vi "UI (Experienced).vi"() -> ()   [LabVIEW 2017, in "UI.lvlib"]
doc: "The Queued Message Handler of a Worker."
uses:
  UI.lvlib
  _support/Analysis Window Type.ctl
  _support/UI State.ctl
  1af51285-6659-428e-9c15-de70f1a207c9.vi
  1756710f-d813-4077-a3f9-6f06171a4225.vi
  b1498353-a107-4479-98d0-7e76c0451ff6.vi
  242d01f8-d211-4c25-bb6c-8191a2acbe42.vi
  da0d510b-1f54-4e49-9d1f-893e7e8abfcf.vi
  e403ca69-710b-4b23-8527-f02bfa86df9b.vi
  <userlib>/_NEVSTOP/Communicable State Machine(CSM)/AdvanceAPI/CSM - Revert Arguments-Safe String.vi
  <userlib>/_NEVSTOP/Communicable State Machine(CSM)/_Shared/Trim Single-line Text.vi
  <userlib>/_NEVSTOP/Communicable State Machine(CSM)/AdvanceAPI/CSM - Make String Arguments Safe.vi
  <userlib>/_NEVSTOP/Communicable State Machine(CSM)/AdvanceAPI/CSM - Break Down Multiple States String.vi
  <userlib>/_NEVSTOP/Communicable State Machine(CSM)/AdvanceAPI/CSM - Keywords.vi
  <userlib>/_NEVSTOP/Communicable State Machine(CSM)/addons/INI-Static-Variable-Support/_Support/instances/_CSM - Read File Logger Configuration - v1.0.vi
  <userlib>/_NEVSTOP/Communicable State Machine(CSM)/addons/API-String-Arugments-Support/_Support/Convert API String Arguments to Data(variant).vi
  <userlib>/_NEVSTOP/Communicable State Machine(CSM)/addons/API-String-Arugments-Support/_Support/Query Data as API String Arguments(variant).vi
  <userlib>/_NEVSTOP/Communicable State Machine(CSM)/addons/MassData-Parameter/_support/FGV-MassData(lvlibp).vi
  <userlib>/_NEVSTOP/Communicable State Machine(CSM)/_Polymophic/Add State(s) to Queue By BOOL(Element).vi
  <userlib>/_NEVSTOP/Communicable State Machine(CSM)/_Polymophic/CSM - Replace Marks in Messages.vi
  Acquisition/Acquisition.lvlib
  Logging/Logging.lvlib
  <userlib>/_NEVSTOP/Communicable State Machine(CSM)/Communicable State Machine.lvlib
  <userlib>/_NEVSTOP/Communicable State Machine(CSM)/addons/MassData-Parameter/CSM MassData Parameter Support.lvlib
  <userlib>/_NEVSTOP/Communicable State Machine(CSM)/addons/INI-Static-Variable-Support/INI-Static-Variable-Support.lvlib
  Algorithm/Algorithm.lvlib
  <userlib>/_NEVSTOP/Communicable State Machine(CSM)/addons/Logger/CSM File Logger.lvlib
  <userlib>/_NEVSTOP/Communicable State Machine(CSM)/addons/Watchdog/CSM Watchdog.lvlib
  <userlib>/_NEVSTOP/Communicable State Machine(CSM)/_Polymophic/Build Synchronous Message with Arguments.vi
panel:
  out "WaveformGraph":waveform(dbl)[](graph)
  in  "Analysis Window 1":T1
  out "AnalysisWnd 1":cluster{"f0":dbl, "df":dbl, "magnitude":dbl[]}[](graph)
  in  "Analysis Window 2":T1
  out "AnalysisWnd 2":cluster{"f0":dbl, "df":dbl, "magnitude":dbl[]}[](graph)
  in  "Settings":bool
  in  "Start":bool
  in  "Stop":bool
  out "Status":string
  in  "Exit":bool
  # "Continuous Measurement and Data Logger - CSM Version"
  # "Experienced Example"
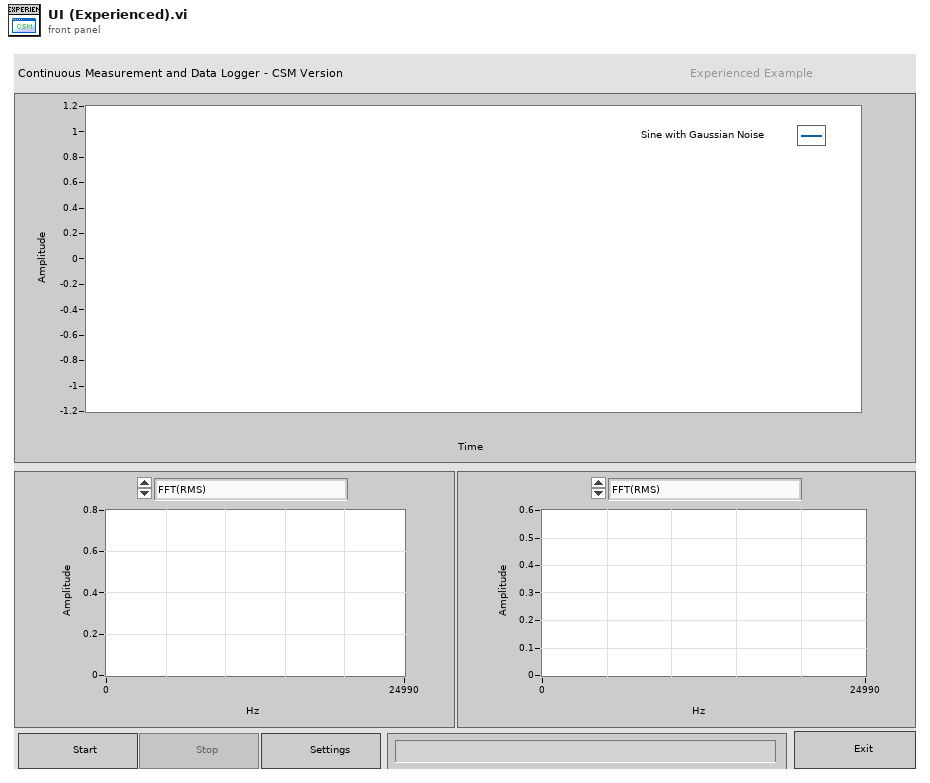
[diagram p1: front panel]
types:
  T1 = typedef "UI.lvlib/Analysis Window Type.ctl" = enum16{"FFT(RMS)", "FFT(Peak)", "Power Spectrum"}
  T2 = cluster{"Enable":bool, "Limit":cluster{"FileSize":i64, "FileNum":i32}, "Timestamp.Format":string, "AutoExit":bool}
  T3 = enum32{"Invalid", "Standard", "Closed", "Hidden", "Minimized", "Maximized"}
  T4 = enum32{"invalid app kind", "Development System", "Run Time System", "Student Edition", "Embedded LabVIEW", "Evaluation", "Custom"}
  T5 = typedef "UI.lvlib/UI State.ctl" = enum16{"Idle", "Acquiring and Logging", "Waiting for Exit", "Waiting for Exit (Acq Stopped)", "Waiting for Exit (Log Stopped)", "Waiting for Stop", "Waiting for Stop (Acq Stopped)", "Waiting for Stop (Log Stopped)"}
  T6 = enum32{"Invalid", "Default", "Floating", "Floating/Auto-Hide", "Modal"}
  T7 = typedef "Communicable State Machine.lvlib/_CSM_Response Source Message.ctl" = cluster{"‘State":string, "’Arguments":string, "’Error":errorcluster}
  T8 = cluster{"Current VI Reference":refnum<vi>, "Close Panel on Exit?":bool}
  T9 = cluster{"Core":cluster{"Current VI Reference":refnum<vi>, "Close Panel on Exit?":bool}, "UI Refs":cluster{"Start Ref":refnum<vi>, "Stop Ref":refnum<vi>, "Settings Ref":refnum<vi>, "Exit Ref":refnum<vi>, "Status Ref":refnum<vi>, "Data Ref":refnum<vi>, "Data Source Ref":refnum<vi>}, "State":T5, "Relationships":string}
  T10 = cluster{"Start Ref":refnum<vi>, "Stop Ref":refnum<vi>, "Settings Ref":refnum<vi>, "Exit Ref":refnum<vi>, "Status Ref":refnum<vi>, "Data Ref":refnum<vi>, "Data Source Ref":refnum<vi>}
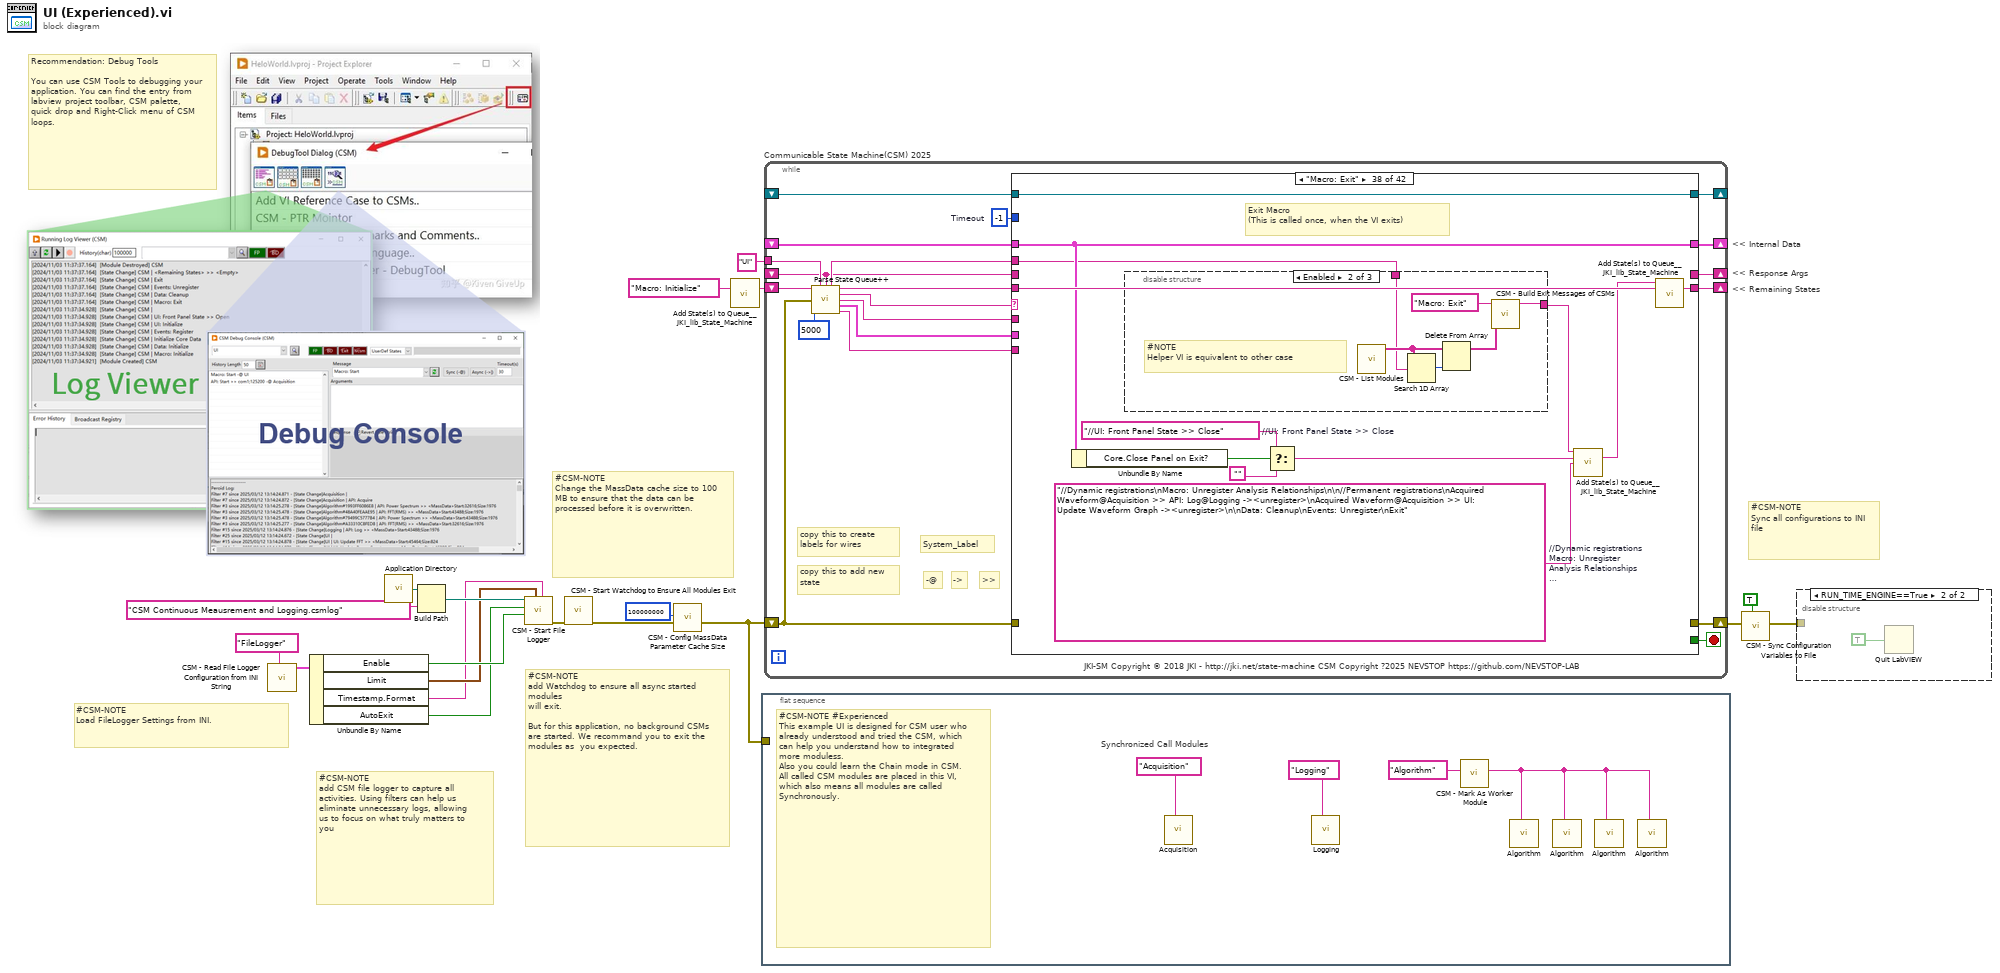
[diagram p0: block diagram]
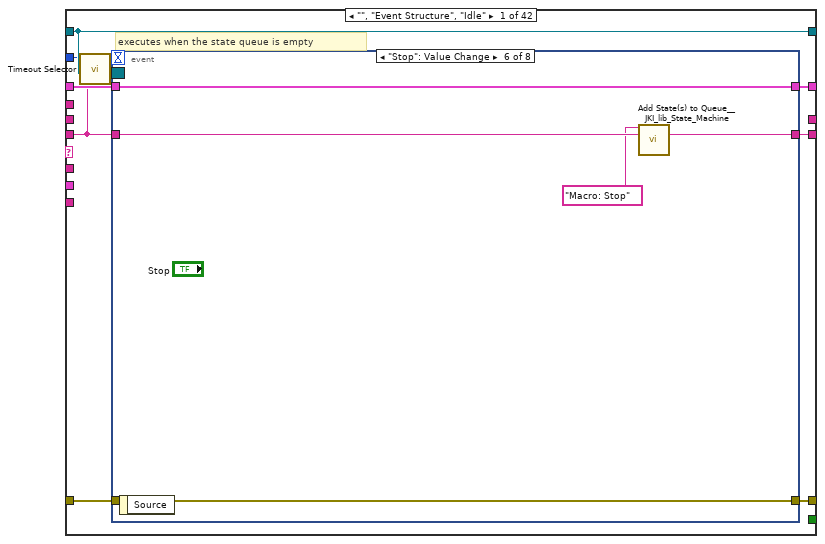
[diagram p3: hidden frame]
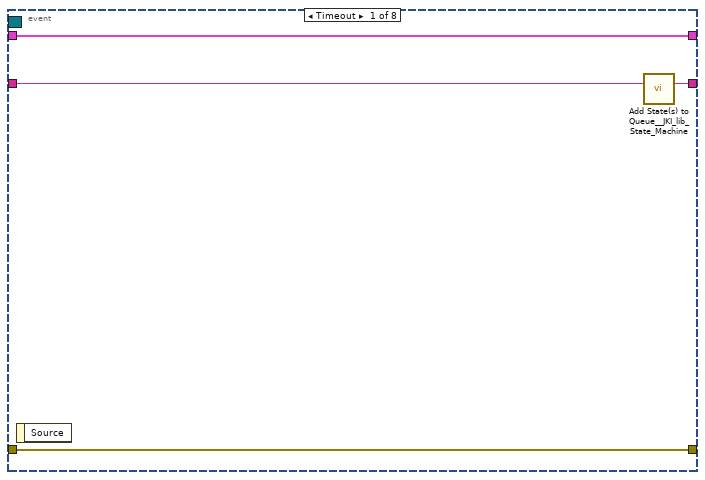
[diagram p4: hidden frame]
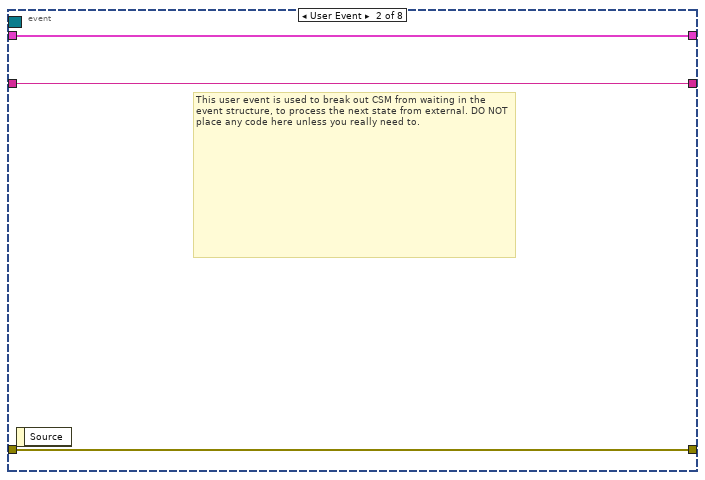
[diagram p5: hidden frame]
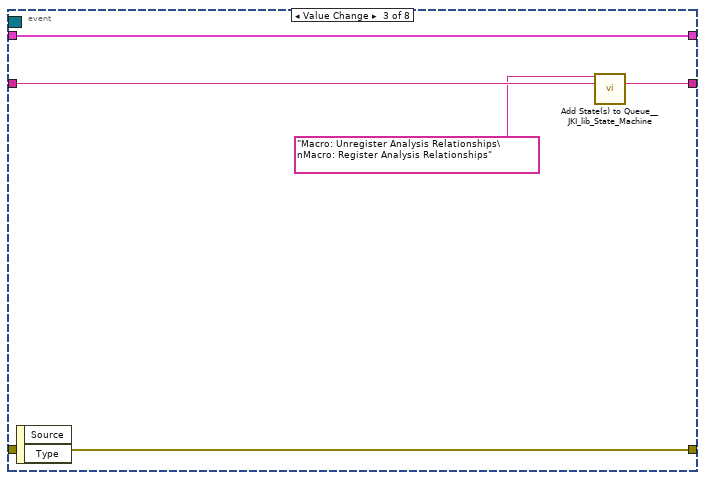
[diagram p6: hidden frame]
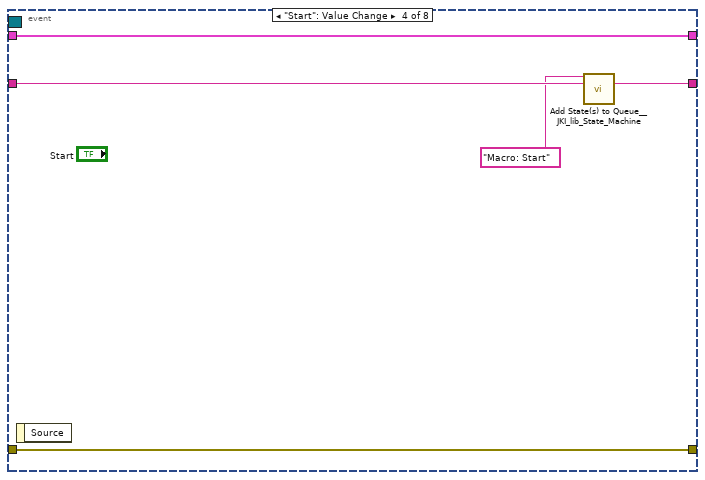
[diagram p7: hidden frame]
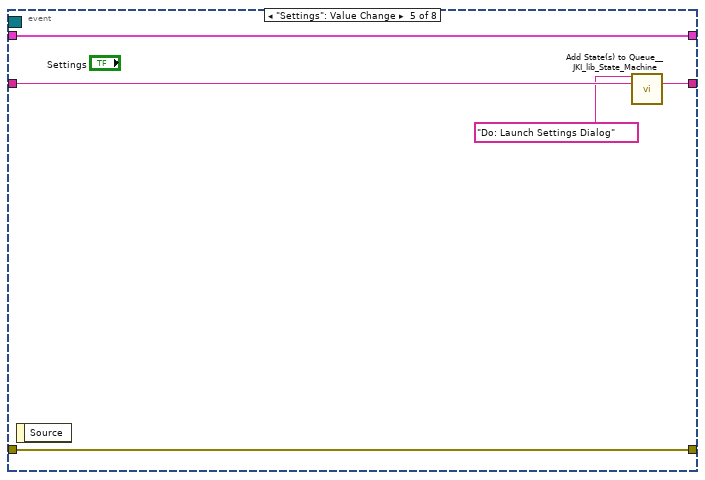
[diagram p8: hidden frame]
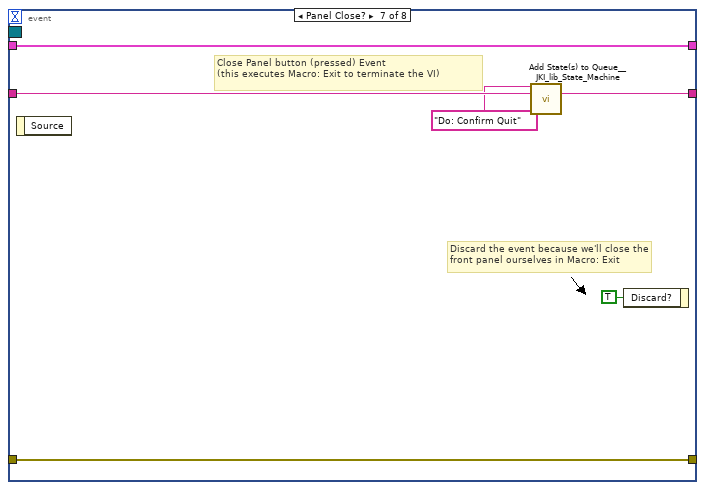
[diagram p9: hidden frame]
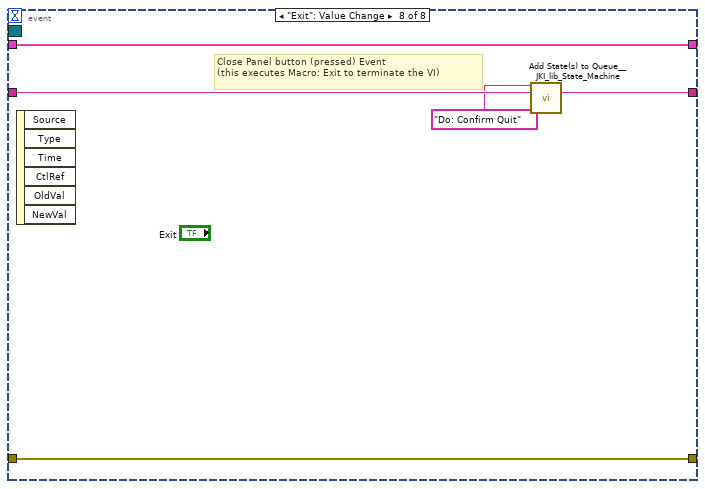
[diagram p10: hidden frame]
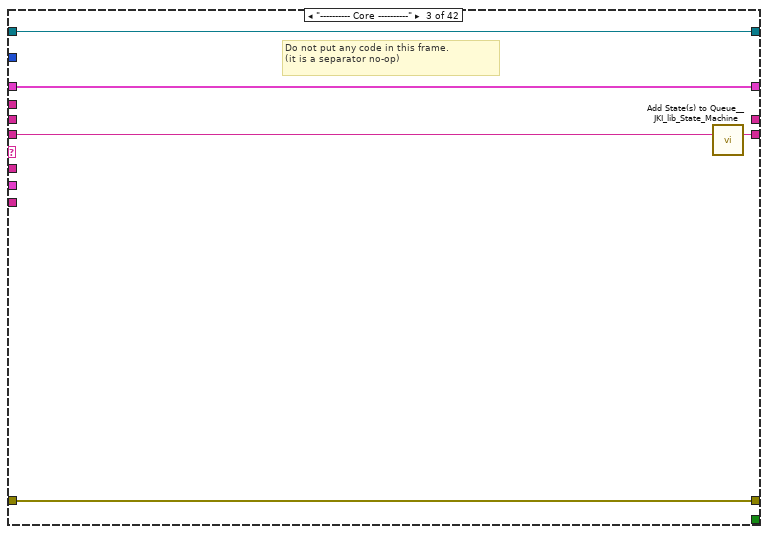
[diagram p12: hidden frame]
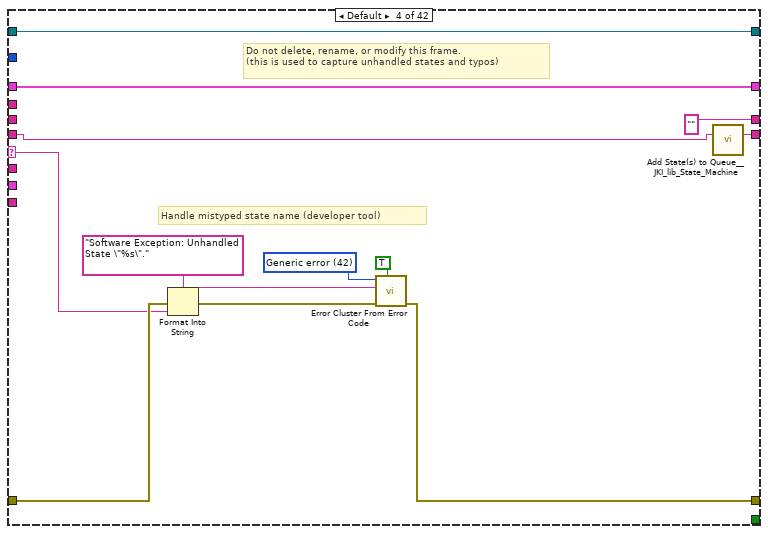
[diagram p13: hidden frame]
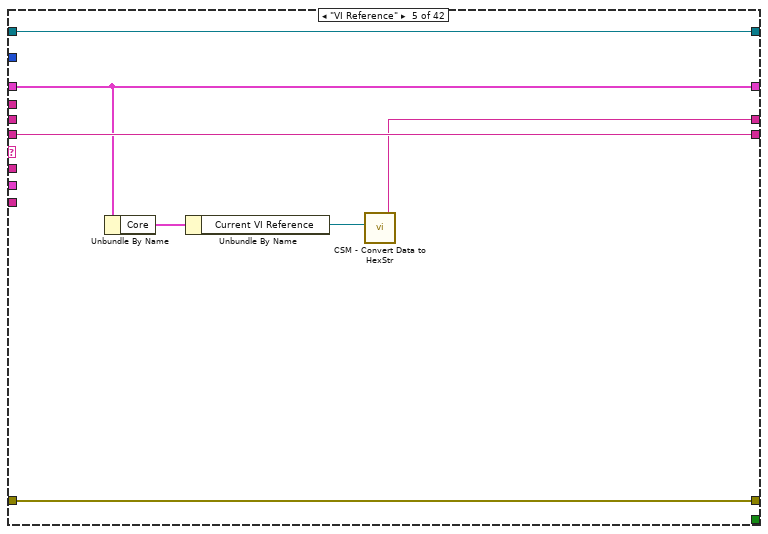
[diagram p14: hidden frame]
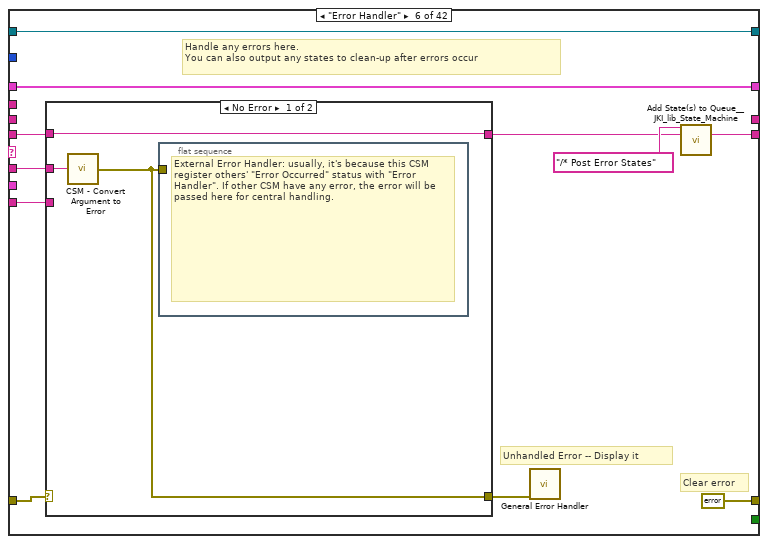
[diagram p15: hidden frame]
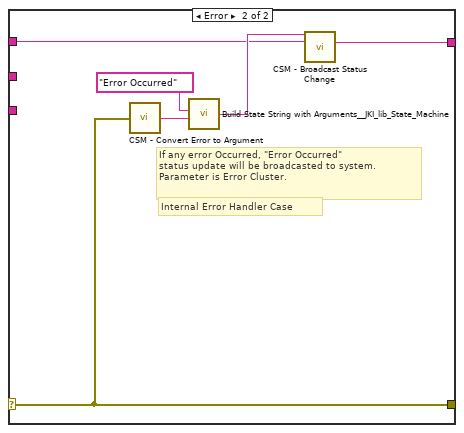
[diagram p16: hidden frame]
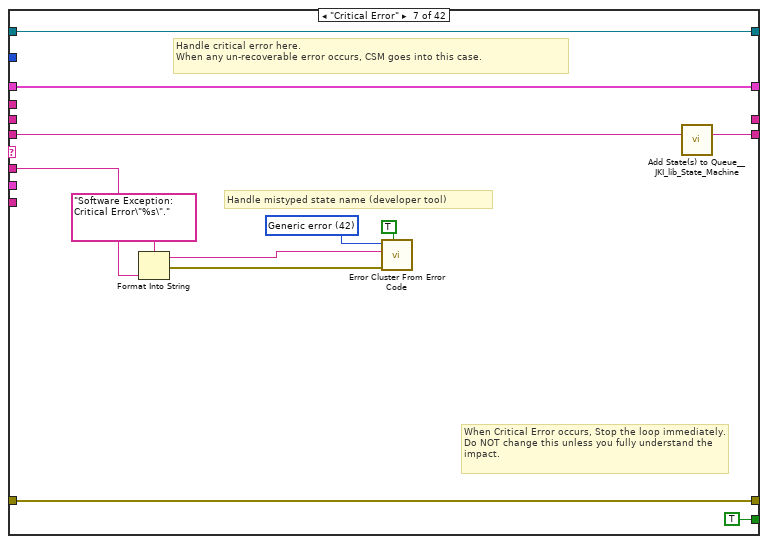
[diagram p17: hidden frame]
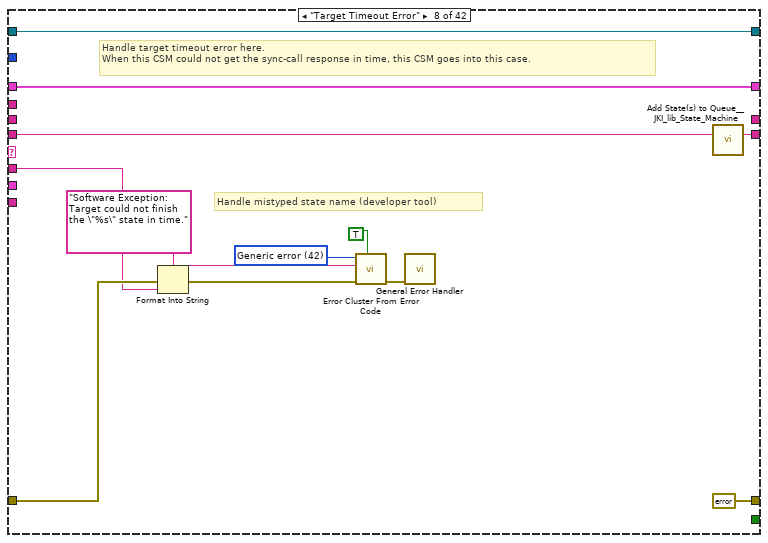
[diagram p18: hidden frame]
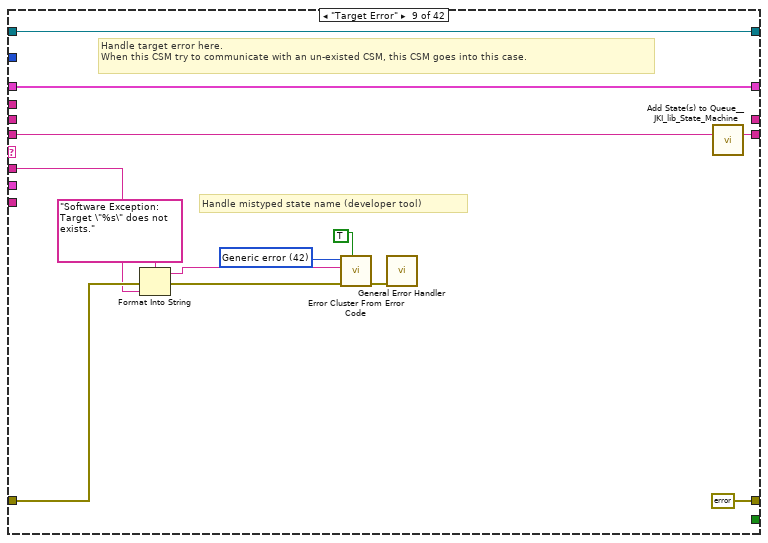
[diagram p19: hidden frame]
diagram:
  # "#CSM-NOTE\nSync all configurations to INI file"
  # "#CSM-NOTE\nChange the MassData cache size to 100 MB to ensure that the data can be processed before it is overwritten."
  # "Recommendation: Debug Tools\n\nYou can use CSM Tools to debugging your application. You can find the entry from labview project toolbar, CSM palette, quick drop and Right-Click menu of CSM loops."
  # "#CSM-NOTE\nLoad FileLogger Settings from INI."
  # "#CSM-NOTE\nadd CSM file logger to capture all activities. Using filters can help us eliminate unnecessary logs, allowing us to focus on what truly matters to you"
  # "#CSM-NOTE\nadd Watchdog to ensure all async started modules\nwill exit. \n\nBut for this application, no background CSMs are started. We recommand you to exit the modules as  you expected."
  # "<< Internal Data"
  # "<< Response Args"
  # "<< Remaining States"
  n1 = call-poly <userlib>:"CSM - Read File Logger Configuration from INI String.vi"("Section Name(\"FileLogger\")"="FileLogger" ("Section Name(\"\" as Default)")) -> ("FileLogger Configuration-v1"=w11:T2)  [unwired: 7 in, 1 out]
  n2 = Unbundle By Name(w11) -> ("Enable"=w10:bool, "Limit"=w9:cluster{"FileSize":i64, "FileNum":i32}, "Timestamp.Format"=w7:string, "AutoExit"=w8:bool)
  n3 = call <vilib>:"Application Directory.vi"() -> ("Application Directory"=w16:path)
  n4 = Build Path(base path=w16, name or relative path="CSM Continuous Meausrement and Logging.csmlog") -> (appended path=w14:path)
  n5 = call <userlib>:"CSM - Start File Logger.vi"("Timestamp Format"=w7, "Log Limit"=w9, "Watchdog? (T)"=w10, "Exit When All Module Exist? (F)"=w8, "Log File Path"=w14) -> ("error out"=w13:errorcluster)  [unwired: 4 in, 2 out]
  n6 = call <userlib>:"CSM - Start Watchdog to Ensure All Modules Exit.vi"("error in (no error)"=w13) -> ("error out"=w5:errorcluster)  [unwired: 10 in]
  n7 = call <userlib>:"CSM - Config MassData Parameter Cache Size.vi"("Error in"=w5, "Size (50M)"=100000000 ("size(1M)")) -> ("Error out"=w4:errorcluster)  [unwired: 9 in]
  n8 = call <vilib>:"Add State(s) to Queue__JKI_lib_State_Machine.vi"("State(s) in (\"\")"="Macro: Initialize") -> ("States Out"=w17:string)  [unwired: 14 in]
  n9 = flat-sequence {
    tunnel: w4 -> [_]
    frame #0 {
      # "#CSM-NOTE #Experienced\nThis example UI is designed for CSM user who already understood and tried the CSM, which can help you understand how to integrated more moduless.\nAlso you could learn the Chain mode in CSM.\nAll called CSM modules are placed in this VI, which also means all modules are called  Synchronously."
      # "Synchronized Call Modules"
      n10 = call "Acquisition.vi"("Name(\"\" to use uuid)"="Acquisition" ("Name(\"\" to use uuid)")) -> ()  [unwired: 11 in]
      n11 = call "Logging.vi"("Name(\"\" to use uuid)"="Logging" ("Name(\"\" to use uuid)")) -> ()  [unwired: 11 in]
      n12 = call <userlib>:"CSM - Mark As Worker Module.vi"("CSM Name"="Algorithm" ("Name(\"\" to use uuid)")) -> ("CSM Name (Marked As Worker)"=w21:string)  [unwired: 9 in]
      n13 = call "Algorithm.vi"("Name(\"\" to use uuid)"=w21) -> ()  [unwired: 11 in]
      n14 = call "Algorithm.vi"("Name(\"\" to use uuid)"=w21) -> ()  [unwired: 11 in]
      n15 = call "Algorithm.vi"("Name(\"\" to use uuid)"=w21) -> ()  [unwired: 11 in]
      n16 = call "Algorithm.vi"("Name(\"\" to use uuid)"=w21) -> ()  [unwired: 11 in]
    }
  }
  n17 = while "Communicable State Machine(CSM) 2025" {
    shift-right: [w39] -> _
    shift-left: _ -> [w38]
    shift-right: [w41] -> w2
    shift-left: w4 -> [w36]
    shift-right: [w40] -> _
    shift-left: w17 -> [w42]
    tunnel: "UI" ("Name(\"\" to use uuid)") -> [w31]
    shift-right: [w34] -> _
    shift-left: _ -> [w26]
    shift-right: [w33] -> _
    shift-left: _ -> [w32]
    stop <- w24 stop-if-true
    w37 = -1  # Timeout
    # "JKI-SM Copyright © 2018 JKI - http://jki.net/state-machine CSM Copyright ?2025 NEVSTOP https://github.com/NEVSTOP-LAB"
    # "copy this to add new state"
    # ">>"
    # "->"
    # "-@"
    # "copy this to create labels for wires"
    # "System_Label"
    n18 = call <userlib>:"Parse State Queue++.vi"("State Queue"=w42, "Name (\"\" to Use UUID)"=w31, "Response Arguments"=w26, "Previous Error"=w36, "Response Timeout (-2 Use Global Settings)"=5000 ("Response Timeout(1000ms)")) -> ("Name Used"=w27:string, "Remaining States"=w43:string, "Current State"=w30:string, "Arguments"=w25:string, "Additional Information"=w29:T7, "Source CSM"=w28:string)  [unwired: 5 in]
    n19 = case shown="\"Macro: Exit\"" w30 {
      selector: w30 -> [_ _ _ w102 _ _ _ _ _ _ _ _ _ _ _ _ _ _ _ _ _ _ _ _ _ _ _ _ _ _ _ _ _ _ _ _ _ _ _ _ _ _]
      tunnel: w43 -> [w44 w93 w99 w106 w118 w123 w149 w159 w172 w180 w184 w199 w206 w211 w220 w226 w233 w240 w245 w251 w255 w261 w281 w295 w308 w316 w332 w406 w415 w428 w435 w440 w447 w455 w463 w474 w485 w503 w528 w534 w542 w580]
      tunnel: w25 -> [_ _ _ _ _ w121 w142 w155 w168 _ _ _ _ _ _ w224 w230 _ _ _ _ _ _ _ _ w311 w326 w401 w419 w425 w432 _ _ _ _ _ _ _ _ w529 _ _]
      tunnel: w38 -> [w51 w92 w96 w104 w117 w129 w150 w157 w170 w179 w183 w192 w204 w208 _ w223 w231 w235 w242 w250 w254 w258 w267 w285 w298 w314 w328 w404 w421 w427 w434 w437 w444 w458 w470 w477 w481 w501 w525 w531 w535 w575]
      tunnel: [w50 w94 w97 w108 w119 errorcluster {"status"=FALSE, "code"=0, "source"=""} ("error out") w151 errorcluster {"status"=FALSE, "code"=0, "source"=""} ("error out") errorcluster {"status"=FALSE, "code"=0, "source"=""} ("error out") w181 w185 w196 w203 w209 w214 w222 w229 w236 w243 w246 w253 w259 w279 w296 w309 w312 w329 w398 w417 w424 w431 w438 w445 w459 w472 w480 w489 _ w526 w532 w536 _] -> w41
      tunnel: w36 -> [w49 w94 w97 w107 w119 w127 w151 w160 w173 w181 w185 w196 w203 w209 w214 _ _ w237 w243 _ w256 w259 w279 w296 w309 w313 w330 _ _ _ _ w438 w445 w459 w472 w480 w489 _ w526 w532 _ _]
      tunnel: [w52 w93 w98 w105 w118 w125 w148 w158 w171 w180 w184 w198 w205 w210 w219 w226 w233 w239 w244 w251 w255 w260 w280 w295 w308 w315 w331 w406 w416 w428 w435 w439 w446 w456 w464 w475 w486 w502 w527 w533 w542 w573] -> w40
      tunnel: [_ _ _ _ _ _ TRUE _ _ _ _ _ TRUE _ _ _ _ _ _ _ _ _ _ _ _ _ _ _ _ _ _ _ _ _ _ _ _ _ _ _ _ _] -> w24
      tunnel: [w48 w92 w96 w104 w117 w129 w150 w157 w170 w179 w183 w197 w204 w208 w213 w221 w227 w235 w242 w250 w254 w258 w266 w285 w298 w314 w328 w404 w421 w427 w434 w437 w444 w454 w461 w476 w487 w501 w525 w531 w535 w574] -> w39
      tunnel: w37 -> [w46 _ _ _ _ _ _ _ _ _ _ _ _ _ _ _ _ _ _ _ _ _ _ _ _ _ _ _ _ _ _ _ _ _ _ _ _ _ _ _ _ _]
      tunnel: w28 -> [_ _ _ _ _ w120 _ _ _ _ _ _ _ _ _ _ _ _ _ _ _ _ _ _ _ _ _ _ _ _ _ _ _ _ _ _ _ _ _ _ _ _]
      tunnel: w29 -> [_ _ _ _ _ _ _ _ _ _ _ _ _ _ _ _ _ _ _ _ _ _ _ _ _ _ _ _ _ _ _ _ _ _ _ _ _ _ _ _ _ _]
      tunnel: [_ _ _ "" w113 _ _ _ _ _ _ _ _ _ _ _ w228 _ _ _ _ _ _ _ _ _ _ _ _ _ _ _ _ _ _ _ _ _ _ _ _ _] -> w34
      tunnel: [w47 w91 w95 w100 w116 w128 w140 w154 w167 w178 w182 w186 w201 w207 w217 w225 w232 w234 w241 w249 w252 w257 w278 w294 w307 w310 w325 w405 w420 w426 w433 w436 w443 w457 w471 w479 w488 w494 w524 w530 w543 w579] -> w33
      tunnel: w32 -> [w47 w91 w95 w100 w116 w128 w140 w154 w167 w178 w182 w186 w201 w207 w217 w225 w232 w234 w241 _ w252 w257 w278 w294 w307 w310 w325 w405 w420 w426 w433 w436 w443 w457 w471 w479 w488 w494 w524 w530 w543 w579]
      tunnel: w27 -> [_ _ _ _ _ _ _ _ _ _ _ _ _ _ _ _ _ _ _ w248 _ _ _ _ _ _ _ _ _ _ _ _ _ _ _ _ _ w492 _ _ w538 _]
      tunnel: w26 -> [_ _ _ _ _ _ _ _ _ _ _ _ _ _ _ _ _ _ _ _ _ _ _ _ _ _ _ _ _ _ _ _ _ _ _ _ _ _ _ _ _ _]
      frame "", "Event Structure", "Idle" {
        # "executes when the state queue is empty"
        n20 = call <userlib>:"Timeout Selector.vi"("Remaining States"=w44, "Timeout Expected"=w46) -> ("Timeout"=w45:i32)  [unwired: 5 in]
        n21 = event shown="[5] \"Stop\": Value Change" {
          selector: w47 -> [_ _ _ _ _ _ _ _]
          dyn-events: _ -> [_ _ _ _ _ _ _ _]
          timeout: w45 -> [_ _ _ _ _ _ _ _]
          tunnel: w44 -> [w56 w58 w61 w66 w71 w76 w85 w90]
          tunnel: [w55 w58 w62 w67 w72 w77 w84 w89] -> w52
          tunnel: w51 -> [w53 w59 w63 w68 w73 w78 w82 w87]
          tunnel: [w54 w57 w64 w69 w74 w79 w83 w88] -> w50
          tunnel: w49 -> [w54 w57 w64 w69 w74 w79 w83 w88]
          tunnel: [w53 w59 w63 w68 w73 w78 w82 w87] -> w48
          event Timeout {
            n22 = event-data() -> ()  [unwired: 1 in, 1 out]
            n23 = call <vilib>:"Add State(s) to Queue__JKI_lib_State_Machine.vi"("State(s) in (\"\")"=w56) -> ("States Out"=w55:string)  [unwired: 14 in]
          }
          event User Event {
            # "This user event is used to break out CSM from waiting in the event structure, to process the next state from external. DO NOT place any code here unless you really need to."
            n24 = event-data() -> ()  [unwired: 1 in, 1 out]
          }
          event Value Change {
            n25 = event-data() -> ()  [unwired: 1 in, 2 out]
            n26 = call <vilib>:"Add State(s) to Queue__JKI_lib_State_Machine.vi"("State(s) in Front (\"\")"="Macro: Unregister Analysis Relationships\nMacro: Register Analysis Relationships" ("State(s) in Front (\"\")"), "State(s) in (\"\")"=w61) -> ("States Out"=w62:string)  [unwired: 13 in]
          }
          event "Start": Value Change {
            n27 = event-data() -> ()  [unwired: 1 in, 1 out]
            n28 = call <vilib>:"Add State(s) to Queue__JKI_lib_State_Machine.vi"("State(s) in Front (\"\")"="Macro: Start" ("State(s) in Front (\"\")"), "State(s) in (\"\")"=w66) -> ("States Out"=w67:string)  [unwired: 13 in]
          }
          event "Settings": Value Change {
            n29 = event-data() -> ()  [unwired: 1 in, 1 out]
            n30 = call <vilib>:"Add State(s) to Queue__JKI_lib_State_Machine.vi"("State(s) in Front (\"\")"="Do: Launch Settings Dialog" ("State(s) in Front (\"\")"), "State(s) in (\"\")"=w71) -> ("States Out"=w72:string)  [unwired: 13 in]
          }
          event "Stop": Value Change {
            n31 = event-data() -> ()  [unwired: 1 in, 1 out]
            n32 = call <vilib>:"Add State(s) to Queue__JKI_lib_State_Machine.vi"("State(s) in Front (\"\")"="Macro: Stop" ("State(s) in Front (\"\")"), "State(s) in (\"\")"=w76) -> ("States Out"=w77:string)  [unwired: 13 in]
          }
          event Panel Close? {
            # "Discard the event because we'll close the front panel ourselves in Macro: Exit"
            # "Close Panel button (pressed) Event\n(this executes Macro: Exit to terminate the VI)"
            n33 = event-data() -> ()  [unwired: 1 in, 1 out]
            n34 = call <vilib>:"Add State(s) to Queue__JKI_lib_State_Machine.vi"("State(s) in Front (\"\")"="Do: Confirm Quit", "State(s) in (\"\")"=w85) -> ("States Out"=w84:string)  [unwired: 13 in]
            n35 = event-data("Discard?"=TRUE) -> ()  [unwired: 1 in, 1 out]
          }
          event "Exit": Value Change {
            # "Close Panel button (pressed) Event\n(this executes Macro: Exit to terminate the VI)"
            n36 = event-data() -> ()  [unwired: 1 in, 6 out]
            n37 = call <vilib>:"Add State(s) to Queue__JKI_lib_State_Machine.vi"("State(s) in Front (\"\")"="Do: Confirm Quit", "State(s) in (\"\")"=w90) -> ("States Out"=w89:string)  [unwired: 13 in]
          }
        }
      }
      frame "CSM Documentation" {
        # "CSM Documentation"
        # "State Syntax:\nStateCategory: State >> Argument -@ CSMName\nStateCategory: State >> Argument -> CSMName\n\nLine Terminator: Line feed"
        # "Commenting:\nTo add a comment use \"//\" or \"#\" and all text to the right will be ignored\nCommenting Example:\nUI: Initialize // This initializes the UI\n// Another comment line"
        # "Example:\nUI: Help >> About -@Main\nUI: Help >> About ->Main\n\nWhere \"UI\" is the state category\nWhere \"Help\" is the state\nWhere \"About\" is the argument\nWhere \"Main\" is the Name of CSM,which actually run the \"UI: Help >> About\"\n\n    \"-@\" stands for sync state. Current CSM will wait until the state is finished. \n            - if \"Main\" named CSM does not exist, \"Target Error\" will occur.\n            - if \"Main\" named CSM is in another sync remote state, \"Target Busy Error\" will occur.\n            - if \"Main\" named CSM could not finish the state in time, \"Target Timeout Error\" will occur.\n            - if everything is right. \"Response\" will occur with Argument back from \"Main\" named CSM. \n\n    \"->\" stands for async state. Current CSM will post the state and continue to next state in next iteration.\n            - if \"Main\" named CSM does not exist, \"Target Error\" will occur.\n            - if everything is right. \"Async Message Posted\" will occur.\n            - After State is finished. Caller will receive a \"Async Response\" state from callee.\n\nWhen duplicated name is used for multiple CSM module or some framework problem happens, \"Critical Error\" will occur."
      }
      frame "---------- Core ----------" {
        # "Do not put any code in this frame.\n(it is a separator no-op)"
        n38 = call <vilib>:"Add State(s) to Queue__JKI_lib_State_Machine.vi"("State(s) in (\"\")"=w99) -> ("States Out"=w98:string)  [unwired: 14 in]
      }
      frame Default {
        w111 = 42 items=["No error", "Argument error", "Memory is full", "Out of zone", "End of file", "File already open", "Generic file I/O error", "File not found", "File permission error", "Disk is full", "Duplicate path", "Too many files open", "System feature not enabled", "Resource file not found", "Cannot add resource", "Resource not found", "Image not found", "Image memory error", "Pen does not exist", "Config type invalid", "Config token not found", "Config parse error", "Config memory error", "Bad external code format", "Bad external code offset", "External code not present", "Null window", "Destroy window error", "Null menu", "Print aborted", "Bad print record", "Print driver error", "Windows error during printing", "Memory error during printing", "Print dialog error", "Generic print error", "Invalid device refnum", "Device not found", "Device parameter error", "Device unit error", "Cannot open device", "Device call aborted", "Generic error", "Cancelled by user", "Object ID too low", "Object ID too high", "Object not in heap", "Unknown heap", "Unknown object (invalid DefProc)", "Unknown object (DefProc not in table)", "Message out of range", "Invalid (null) method", "Unknown message", "Manager call not supported", "Bad address", "Network operation in progress", "Network operation timed out", "Connection is busy", "Network attribute not supported", "Network error", "Address in use", "System out of memory", "Connection aborted", "Connection refused", "Not connected", "Already connected", "Connection closed", "Initialization error (interapplication manager)", "Bad occurrence", "Wait on unbound occurrence handler", "Occurrence queue overflow", "Datalog type conflict", "Unused", "Unrecognized type (interapplication manager)", "Memory corrupt", "Failed to make temporary DLL", "Old CIN version", "Drag socket not found", "Failed to load drop-object", "Failed to register OLE object", "Failed to release OLE object", "Format specifier type mismatch", "Unknown format specifier", "Too few format specifiers", "Too many format specifiers", "Scan failed", "Newer CIN version", "Error converting to variant", "Runtime menu error", "Password tampered", "Variant attribute not found", "Incompatible variant data type", "Event data is not available", "Event Store is not present", "Occurrence is not found", "Event Queue is not created", "Event info is not available", "Refnum passed is NULL", "Error retrieving Class GUID", "Error retrieving CoClass GUID", "Error retrieving TypeLib GUID.", "Bad built application magic bytes.", "Specific driver is different from the specific driver associated with the Logical Name.", "There is no session opened to the class driver.", "Max Error", "MAX - Error with config objects", "MAX - Error loading configuration", "MAX - Group not supported"]
        # "Do not delete, rename, or modify this frame.\n(this is used to capture unhandled states and typos)"
        # "Handle mistyped state name (developer tool)"
        n39 = Format Into String(format string="Software Exception: Unhandled State \"%s\"." ("message"), error in=w107, w102) -> (resulting string=w110:string, error out=w109:errorcluster)  [unwired: 1 in]
        n40 = call <vilib>:"Error Cluster From Error Code.vi"("show call chain? (False)"=TRUE, "error in (no error)"=w109, "error message (\"\")"=w110, "error code (0)"=w111) -> ("error out"=w108:errorcluster)  [unwired: 5 in]
        n41 = call <vilib>:"Add State(s) to Queue__JKI_lib_State_Machine.vi"("State(s) in (\"\")"=w106) -> ("States Out"=w105:string)  [unwired: 14 in]
      }
      frame "VI Reference" {
        n42 = Unbundle By Name(w117) -> ("Core"=w115:T8)
        n43 = Unbundle By Name(w115) -> ("Current VI Reference"=w114:refnum<vi>)
        n44 = call <userlib>:"CSM - Convert Data to HexStr.vi"("Variant"=w114) -> ("HEX String (0-9,A-F)"=w113:string)  [unwired: 8 in]
      }
      frame "Error Handler" {
        # "Unhandled Error -- Display it"
        # "Handle any errors here.\nYou can also output any states to clean-up after errors occur"
        # "Clear error"
        n45 = case shown="No Error" w127 {
          selector: w127 -> [_ w134]
          tunnel: [w132 w136] -> w124
          tunnel: w123 -> [w132 w135]
          tunnel: [w131 w134] -> w122
          tunnel: w121 -> [w133 _]
          tunnel: w120 -> [_ _]
          frame No Error {
            n46 = call <userlib>:"CSM - Convert Argument to Error.vi"("Argument"=w133) -> ("Error"=w131:errorcluster)  [unwired: 4 in]
            n47 = flat-sequence {
              tunnel: w131 -> [_]
              frame #0 {
                # "External Error Handler: usually, it's because this CSM register others' \"Error Occurred\" status with \"Error Handler\". If other CSM have any error, the error will be passed here for central handling."
              }
            }
          }
          frame Error {
            # "Internal Error Handler Case"
            # "If any error Occurred, \"Error Occurred\" \nstatus update will be broadcasted to system.\nParameter is Error Cluster."
            n48 = call <userlib>:"CSM - Convert Error to Argument.vi"("Error"=w134) -> ("Argument"=w138:string)  [unwired: 4 in]
            n49 = call <vilib>:"Build State String with Arguments__JKI_lib_State_Machine.vi"("Arguments (\"\")"=w138, "State"="Error Occurred" ("Status with Arguments")) -> ("State with Arguments"=w137:string)  [unwired: 4 in]
            n50 = call <userlib>:"CSM - Broadcast Status Change.vi"("Status With Arguments"=w137, "State Queue"=w135) -> ("Remaining States"=w136:string)  [unwired: 13 in]
          }
        }
        n51 = call <vilib>:"General Error Handler.vi"("error in (no error)"=w122) -> ()  [unwired: 10 in, 5 out]
        n52 = call <vilib>:"Add State(s) to Queue__JKI_lib_State_Machine.vi"("State(s) in Front (\"\")"="/* Post Error States", "State(s) in (\"\")"=w124) -> ("States Out"=w125:string)  [unwired: 13 in]
      }
      frame "Critical Error" {
        w146 = 42 items=["No error", "Argument error", "Memory is full", "Out of zone", "End of file", "File already open", "Generic file I/O error", "File not found", "File permission error", "Disk is full", "Duplicate path", "Too many files open", "System feature not enabled", "Resource file not found", "Cannot add resource", "Resource not found", "Image not found", "Image memory error", "Pen does not exist", "Config type invalid", "Config token not found", "Config parse error", "Config memory error", "Bad external code format", "Bad external code offset", "External code not present", "Null window", "Destroy window error", "Null menu", "Print aborted", "Bad print record", "Print driver error", "Windows error during printing", "Memory error during printing", "Print dialog error", "Generic print error", "Invalid device refnum", "Device not found", "Device parameter error", "Device unit error", "Cannot open device", "Device call aborted", "Generic error", "Cancelled by user", "Object ID too low", "Object ID too high", "Object not in heap", "Unknown heap", "Unknown object (invalid DefProc)", "Unknown object (DefProc not in table)", "Message out of range", "Invalid (null) method", "Unknown message", "Manager call not supported", "Bad address", "Network operation in progress", "Network operation timed out", "Connection is busy", "Network attribute not supported", "Network error", "Address in use", "System out of memory", "Connection aborted", "Connection refused", "Not connected", "Already connected", "Connection closed", "Initialization error (interapplication manager)", "Bad occurrence", "Wait on unbound occurrence handler", "Occurrence queue overflow", "Datalog type conflict", "Unused", "Unrecognized type (interapplication manager)", "Memory corrupt", "Failed to make temporary DLL", "Old CIN version", "Drag socket not found", "Failed to load drop-object", "Failed to register OLE object", "Failed to release OLE object", "Format specifier type mismatch", "Unknown format specifier", "Too few format specifiers", "Too many format specifiers", "Scan failed", "Newer CIN version", "Error converting to variant", "Runtime menu error", "Password tampered", "Variant attribute not found", "Incompatible variant data type", "Event data is not available", "Event Store is not present", "Occurrence is not found", "Event Queue is not created", "Event info is not available", "Refnum passed is NULL", "Error retrieving Class GUID", "Error retrieving CoClass GUID", "Error retrieving TypeLib GUID.", "Bad built application magic bytes.", "Specific driver is different from the specific driver associated with the Logical Name.", "There is no session opened to the class driver.", "Max Error", "MAX - Error with config objects", "MAX - Error loading configuration", "MAX - Group not supported"]
        # "Handle critical error here.\nWhen any un-recoverable error occurs, CSM goes into this case."
        # "When Critical Error occurs, Stop the loop immediately. Do NOT change this unless you fully understand the impact."
        # "Handle mistyped state name (developer tool)"
        n53 = Format Into String(format string="Software Exception: Critical Error\"%s\"." ("message"), w142) -> (resulting string=w145:string, error out=w144:errorcluster)  [unwired: 2 in]
        n54 = call <vilib>:"Error Cluster From Error Code.vi"("show call chain? (False)"=TRUE, "error in (no error)"=w144, "error message (\"\")"=w145, "error code (0)"=w146) -> ()  [unwired: 5 in, 1 out]
        n55 = call <vilib>:"Add State(s) to Queue__JKI_lib_State_Machine.vi"("State(s) in (\"\")"=w149) -> ("States Out"=w148:string)  [unwired: 14 in]
      }
      frame "Target Timeout Error" {
        w163 = 42 items=["No error", "Argument error", "Memory is full", "Out of zone", "End of file", "File already open", "Generic file I/O error", "File not found", "File permission error", "Disk is full", "Duplicate path", "Too many files open", "System feature not enabled", "Resource file not found", "Cannot add resource", "Resource not found", "Image not found", "Image memory error", "Pen does not exist", "Config type invalid", "Config token not found", "Config parse error", "Config memory error", "Bad external code format", "Bad external code offset", "External code not present", "Null window", "Destroy window error", "Null menu", "Print aborted", "Bad print record", "Print driver error", "Windows error during printing", "Memory error during printing", "Print dialog error", "Generic print error", "Invalid device refnum", "Device not found", "Device parameter error", "Device unit error", "Cannot open device", "Device call aborted", "Generic error", "Cancelled by user", "Object ID too low", "Object ID too high", "Object not in heap", "Unknown heap", "Unknown object (invalid DefProc)", "Unknown object (DefProc not in table)", "Message out of range", "Invalid (null) method", "Unknown message", "Manager call not supported", "Bad address", "Network operation in progress", "Network operation timed out", "Connection is busy", "Network attribute not supported", "Network error", "Address in use", "System out of memory", "Connection aborted", "Connection refused", "Not connected", "Already connected", "Connection closed", "Initialization error (interapplication manager)", "Bad occurrence", "Wait on unbound occurrence handler", "Occurrence queue overflow", "Datalog type conflict", "Unused", "Unrecognized type (interapplication manager)", "Memory corrupt", "Failed to make temporary DLL", "Old CIN version", "Drag socket not found", "Failed to load drop-object", "Failed to register OLE object", "Failed to release OLE object", "Format specifier type mismatch", "Unknown format specifier", "Too few format specifiers", "Too many format specifiers", "Scan failed", "Newer CIN version", "Error converting to variant", "Runtime menu error", "Password tampered", "Variant attribute not found", "Incompatible variant data type", "Event data is not available", "Event Store is not present", "Occurrence is not found", "Event Queue is not created", "Event info is not available", "Refnum passed is NULL", "Error retrieving Class GUID", "Error retrieving CoClass GUID", "Error retrieving TypeLib GUID.", "Bad built application magic bytes.", "Specific driver is different from the specific driver associated with the Logical Name.", "There is no session opened to the class driver.", "Max Error", "MAX - Error with config objects", "MAX - Error loading configuration", "MAX - Group not supported"]
        # "Handle target timeout error here.\nWhen this CSM could not get the sync-call response in time, this CSM goes into this case."
        # "Handle mistyped state name (developer tool)"
        n56 = Format Into String(format string="Software Exception: Target could not finish the \"%s\" state in time." ("message"), error in=w160, w155) -> (resulting string=w162:string, error out=w161:errorcluster)  [unwired: 1 in]
        n57 = call <vilib>:"Error Cluster From Error Code.vi"("show call chain? (False)"=TRUE, "error in (no error)"=w161, "error message (\"\")"=w162, "error code (0)"=w163) -> ("error out"=w152:errorcluster)  [unwired: 5 in]
        n58 = call <vilib>:"General Error Handler.vi"("error in (no error)"=w152) -> ()  [unwired: 10 in, 5 out]
        n59 = call <vilib>:"Add State(s) to Queue__JKI_lib_State_Machine.vi"("State(s) in (\"\")"=w159) -> ("States Out"=w158:string)  [unwired: 14 in]
      }
      frame "Target Error" {
        w176 = 42 items=["No error", "Argument error", "Memory is full", "Out of zone", "End of file", "File already open", "Generic file I/O error", "File not found", "File permission error", "Disk is full", "Duplicate path", "Too many files open", "System feature not enabled", "Resource file not found", "Cannot add resource", "Resource not found", "Image not found", "Image memory error", "Pen does not exist", "Config type invalid", "Config token not found", "Config parse error", "Config memory error", "Bad external code format", "Bad external code offset", "External code not present", "Null window", "Destroy window error", "Null menu", "Print aborted", "Bad print record", "Print driver error", "Windows error during printing", "Memory error during printing", "Print dialog error", "Generic print error", "Invalid device refnum", "Device not found", "Device parameter error", "Device unit error", "Cannot open device", "Device call aborted", "Generic error", "Cancelled by user", "Object ID too low", "Object ID too high", "Object not in heap", "Unknown heap", "Unknown object (invalid DefProc)", "Unknown object (DefProc not in table)", "Message out of range", "Invalid (null) method", "Unknown message", "Manager call not supported", "Bad address", "Network operation in progress", "Network operation timed out", "Connection is busy", "Network attribute not supported", "Network error", "Address in use", "System out of memory", "Connection aborted", "Connection refused", "Not connected", "Already connected", "Connection closed", "Initialization error (interapplication manager)", "Bad occurrence", "Wait on unbound occurrence handler", "Occurrence queue overflow", "Datalog type conflict", "Unused", "Unrecognized type (interapplication manager)", "Memory corrupt", "Failed to make temporary DLL", "Old CIN version", "Drag socket not found", "Failed to load drop-object", "Failed to register OLE object", "Failed to release OLE object", "Format specifier type mismatch", "Unknown format specifier", "Too few format specifiers", "Too many format specifiers", "Scan failed", "Newer CIN version", "Error converting to variant", "Runtime menu error", "Password tampered", "Variant attribute not found", "Incompatible variant data type", "Event data is not available", "Event Store is not present", "Occurrence is not found", "Event Queue is not created", "Event info is not available", "Refnum passed is NULL", "Error retrieving Class GUID", "Error retrieving CoClass GUID", "Error retrieving TypeLib GUID.", "Bad built application magic bytes.", "Specific driver is different from the specific driver associated with the Logical Name.", "There is no session opened to the class driver.", "Max Error", "MAX - Error with config objects", "MAX - Error loading configuration", "MAX - Group not supported"]
        # "Handle target error here.\nWhen this CSM try to communicate with an un-existed CSM, this CSM goes into this case."
        # "Handle mistyped state name (developer tool)"
        n60 = Format Into String(format string="Software Exception: Target \"%s\" does not exists." ("message"), error in=w173, w168) -> (resulting string=w175:string, error out=w174:errorcluster)  [unwired: 1 in]
        n61 = call <vilib>:"Error Cluster From Error Code.vi"("show call chain? (False)"=TRUE, "error in (no error)"=w174, "error message (\"\")"=w175, "error code (0)"=w176) -> ("error out"=w166:errorcluster)  [unwired: 5 in]
        n62 = call <vilib>:"General Error Handler.vi"("error in (no error)"=w166) -> ()  [unwired: 10 in, 5 out]
        n63 = call <vilib>:"Add State(s) to Queue__JKI_lib_State_Machine.vi"("State(s) in (\"\")"=w172) -> ("States Out"=w171:string)  [unwired: 14 in]
      }
      frame "Async Response", "Response" {
        # "Handle Async-call Response (\"Async Response\" for ->)"
        # "Handle Sync-call Response (\"Response\" for -@)"
        # "After Message is executed, CSM+ goes to this state for receive the response. \n    For Async Message(->), \"Async Response\" is used. This CSM will goes to \"Async Message Posted\" immediately and receive the \"Async Response\" after the callee finishes the message.\n    For Sync Message(@),  This CSM will wait until the message is done and immediately goes to \"Response\""
      }
      frame "Async Message Posted" {
        # "Handle post action for async message (->)."
        # "After Async Message is posted (->), CSM+ goes to this state for post-action. You can use Argument - State to tell which Async Message is called."
      }
      frame "Initialize Core Data" {
        # "Do not delete, rename, or modify this frame.\n(this is used to determine panel behavior on exit)"
        # "originally closed?"
        # "exe?"
        # "If panel starts closed or is an EXE, then close it when we exit"
        n64 = property class="VI"() -> ("FP.State"=w189:T3)  [unwired: 2 in, 2 out]
        n65 = property class="App"() -> ("App.Kind"=w195:T4)  [unwired: 2 in, 2 out]
        n66 = control-ref of="Current VI Reference"() -> (w190:refnum<vi>)
        n67 = Equal?(x=w189, y=T3."Closed" ("Front Panel Window:State")) -> (x = y?=w187:bool)
        n68 = Equal?(x=w195, y=T4."Run Time System" ("Application:Kind")) -> (x = y?=w193:bool)
        n69 = Or(x=w187, y=w193) -> (x .or. y?=w191:bool)
        n70 = Bundle By Name(cluster=w192, "Core.Current VI Reference"=w190, "Core.Close Panel on Exit?"=w191) -> (w197:T9)
        n71 = call <vilib>:"Add State(s) to Queue__JKI_lib_State_Machine.vi"("State(s) in (\"\")"=w199) -> ("States Out"=w198:string)  [unwired: 14 in]
      }
      frame "Exit" {
        # "Do not put any code in this frame.\n(No errors that occur here will be handled.)"
        n72 = local write "Status"("Exit" ("Exit String")) -> ()
        n73 = call <vilib>:"Add State(s) to Queue__JKI_lib_State_Machine.vi"("State(s) in (\"\")"=w206) -> ("States Out"=w205:string)  [unwired: 14 in]
      }
      frame "---------- Data ----------" {
        # "Do not put any code in this frame.\n(It is a separator no-op. You can make a copy of this frame to create a new Data frame)"
        n74 = call <vilib>:"Add State(s) to Queue__JKI_lib_State_Machine.vi"("State(s) in (\"\")"=w211) -> ("States Out"=w210:string)  [unwired: 14 in]
      }
      frame "Data: Initialize" {
        w212 = ""  # Relationships
        w215 = UI_State."Idle"  # State
        w216 = T10 {"Start Ref"=refnum, "Stop Ref"=refnum, "Settings Ref"=refnum, "Exit Ref"=refnum, "Status Ref"=refnum, "Data Ref"=refnum, "Data Source Ref"=refnum}  # UI Refs
        w218 = T8 {"Current VI Reference"=refnum, "Close Panel on Exit?"=FALSE}  # Core
        # "Initialize the shift-register data, here.\n(data names are defined by what you wire into the bundle function)"
        n75 = Bundle("Core"=w218, "UI Refs"=w216, "State"=w215, "Relationships"=w212) -> (w213:T9)  [unwired: 1 in]
        n76 = call <vilib>:"Add State(s) to Queue__JKI_lib_State_Machine.vi"("State(s) in (\"\")"=w220) -> ("States Out"=w219:string)  [unwired: 14 in]
      }
      frame "Data: Set Configuration" {
        n77 = call "Convert API String Arguments to Data.vim"("Reference Type"=w223, "API String"=w224) -> ("error out"=w222:errorcluster, "Data"=w221:T9)  [unwired: 6 in]
      }
      frame "Data: Get Configuration", "Data: Get Internal Data" {
        n78 = call "Query Data as API String Arguments.vim"("Name"=w230, "Cluster Data"=w231) -> ("error"=w229:errorcluster, "API String"=w228:string, "Cluster Data (dup)"=w227:T9)  [unwired: 7 in]
      }
      frame "Data: Cleanup" {
        # "Cleanup any data and references, here.\n(this is called automatically, by the Macro: Exit)"
        n79 = Unbundle By Name(w235) -> ("Core.Current VI Reference"=w238:refnum<vi>)
        n80 = Close Reference(reference=w238, error in (no error)=w237) -> (error out=w236:errorcluster)
        n81 = call <vilib>:"Add State(s) to Queue__JKI_lib_State_Machine.vi"("State(s) in (\"\")"=w240) -> ("States Out"=w239:string)  [unwired: 14 in]
      }
      frame "---------- Events ----------" {
        # "Do not put any code in this frame.\n(It is a separator no-op. You can make a copy of this frame to create a new UI frame)"
        n82 = call <vilib>:"Add State(s) to Queue__JKI_lib_State_Machine.vi"("State(s) in (\"\")"=w245) -> ("States Out"=w244:string)  [unwired: 14 in]
      }
      frame "Events: Register" {
        # "Register message event to break Waiting in Event structure."
        n83 = call <userlib>:"CSM - Get New State Notifier Event.vi"("Name (\"\" to Use UUID)"=w248) -> ("error out"=w246:errorcluster, "New State Notifier Event"=w247:refnum<user-event>)  [unwired: 9 in]
        n84 = register-events(w247) -> (reference out=w249:refnum<event-registration>)  [unwired: 2 in, 1 out]
      }
      frame "Events: Unregister" {
        n85 = Unregister For Events(event registration refnum=w252, error in=w256) -> (error out=w253:errorcluster)
      }
      frame "---------- UI ----------" {
        # "Do not put any code in this frame.\n(It is a separator no-op. You can make a copy of this frame to create a new UI frame)"
        n86 = call <vilib>:"Add State(s) to Queue__JKI_lib_State_Machine.vi"("State(s) in (\"\")"=w261) -> ("States Out"=w260:string)  [unwired: 14 in]
      }
      frame "UI: Initialize" {
        w262 = cluster{"f0":dbl, "df":dbl, "magnitude":dbl[]}[] [] ("FFT")
        # "Initialize the User Interface, here.\n(this is called automatically, by the Macro: Init)"
        n87 = control-ref of="WaveformGraph"() -> (w270:refnum<vi>)
        n88 = property on="AnalysisWnd 1" class="WFGraph (strict)"("Value"=w262) -> ()  [unwired: 2 in, 2 out]
        n89 = property on="AnalysisWnd 2" class="WFGraph (strict)"("Value"=w262) -> ()  [unwired: 2 in, 2 out]
        n90 = property on="WaveformGraph" class="WFChart (strict)"("History Data"=waveform(dbl)[][] []) -> ()  [unwired: 2 in, 2 out]
        n91 = control-ref of="Start"() -> (w275:refnum<vi>)
        n92 = control-ref of="Stop"() -> (w274:refnum<vi>)
        n93 = control-ref of="Settings"() -> (w276:refnum<vi>)
        n94 = control-ref of="Exit"() -> (w277:refnum<vi>)
        n95 = control-ref of="Status"() -> (w271:refnum<vi>)
        n96 = Bundle By Name(cluster=w267, "UI Refs.Start Ref"=w275, "UI Refs.Stop Ref"=w274, "UI Refs.Settings Ref"=w276, "UI Refs.Exit Ref"=w277, "UI Refs.Status Ref"=w271, "UI Refs.Data Ref"=w270) -> (w266:T9)
        n97 = Build Array(w275, w277, w276) -> (w273:refnum<vi>[])
        n98 = Build Array(w274) -> (w272:refnum<vi>[])
        n99 = local write "Analysis Window 1"(Analysis_Window_Type."FFT(RMS)" ("Analysis Window 1")) -> ()
        n100 = local write "Analysis Window 2"(Analysis_Window_Type."Power Spectrum" ("Analysis Window 2")) -> ()
        n101 = call "Set Enable State on Multiple Controls.vi"("Enable?"=TRUE, "Controls"=w273) -> ()  [unwired: 10 in]
        n102 = call "Set Enable State on Multiple Controls.vi"("Enable?"=FALSE, "Controls"=w272) -> ()  [unwired: 10 in]
        n103 = call <vilib>:"Add State(s) to Queue__JKI_lib_State_Machine.vi"("State(s) in (\"\")"=w281) -> ("States Out"=w280:string)  [unwired: 14 in]
      }
      frame "UI: Update When Start" {
        w283 = cluster{"f0":dbl, "df":dbl, "magnitude":dbl[]}[] [] ("FFT")
        # "Enable: Stop\nDisable: Start, Exit, Settings"
        n104 = property on="AnalysisWnd 1" class="WFGraph (strict)"("Value"=w283) -> ()  [unwired: 2 in, 2 out]
        n105 = property on="AnalysisWnd 2" class="WFGraph (strict)"("Value"=w283) -> ()  [unwired: 2 in, 2 out]
        n106 = property on="WaveformGraph" class="WFChart (strict)"("History Data"=waveform(dbl)[][] []) -> ()  [unwired: 2 in, 2 out]
        n107 = Unbundle By Name(w285) -> ("UI Refs.Stop Ref"=w291:refnum<vi>, "UI Refs.Start Ref"=w290:refnum<vi>, "UI Refs.Exit Ref"=w289:refnum<vi>, "UI Refs.Settings Ref"=w288:refnum<vi>, "UI Refs.Data Source Ref"=w284:refnum<vi>)
        n108 = Build Array(w290, w289, w288, w284) -> (w293:refnum<vi>[])
        n109 = Build Array(w291) -> (w292:refnum<vi>[])
        n110 = call "Set Enable State on Multiple Controls.vi"("Enable?"=TRUE, "Controls"=w292) -> ()  [unwired: 10 in]
        n111 = call "Set Enable State on Multiple Controls.vi"("Enable?"=FALSE, "Controls"=w293) -> ()  [unwired: 10 in]
      }
      frame "UI: Update When Stop" {
        # "Enable: Start, Exit, Settings\nDisable: Stop"
        n112 = Unbundle By Name(w298) -> ("UI Refs.Stop Ref"=w303:refnum<vi>, "UI Refs.Start Ref"=w304:refnum<vi>, "UI Refs.Exit Ref"=w305:refnum<vi>, "UI Refs.Settings Ref"=w306:refnum<vi>, "UI Refs.Data Source Ref"=w297:refnum<vi>)
        n113 = Build Array(w304, w305, w306, w297) -> (w301:refnum<vi>[])
        n114 = Build Array(w303) -> (w302:refnum<vi>[])
        n115 = call "Set Enable State on Multiple Controls.vi"("Enable?"=FALSE, "Controls"=w302) -> ()  [unwired: 10 in]
        n116 = call "Set Enable State on Multiple Controls.vi"("Enable?"=TRUE, "Controls"=w301) -> ()  [unwired: 10 in]
      }
      frame "UI: Cursor Set" {
        # "Argument"
        # "Set and Unset Cursor Busy.\n(Usage: \"UI: Cursor Set >> Busy|Idle\")"
        n117 = disable-structure shown="Default" {
          disable-tunnel: w313 -> [w319 w324]
          disable-tunnel: [w318 w324] -> w312
          disable-tunnel: w311 -> [w317 _]
          frame condition #0 (active) {
            n118 = case shown="\"Busy\"" w317 {
              tunnel: w319 -> [w321 w323]
              tunnel: [w320 w322] -> w318
              frame "Idle", Default {
                n119 = call <vilib>:"Unset Busy.vi"("error in (no error)"=w321) -> ("error out"=w320:errorcluster)  [unwired: 10 in]
              }
              frame "Busy" {
                n120 = call <vilib>:"Set Busy.vi"("error in (no error)"=w323) -> ("error out"=w322:errorcluster)  [unwired: 9 in, 1 out]
              }
            }
          }
          frame condition #1 {
          }
        }
        n121 = call <vilib>:"Add State(s) to Queue__JKI_lib_State_Machine.vi"("State(s) in (\"\")"=w316) -> ("States Out"=w315:string)  [unwired: 14 in]
      }
      frame "UI: Front Panel State" {
        # "Argument"
        # "Set Front Panel Open or Closed\n(Usage: \"UI: Front Panel State >> Open|Close\")"
        n122 = Unbundle By Name(w328) -> ("Core.Current VI Reference"=w327:refnum<vi>)
        n123 = case shown="\"Minimize\", \"Minimized\"" w326 {
          tunnel: w330 -> [w338 w353 w364 w377 w390]
          tunnel: [w340 w354 w366 w379 w392] -> w329
          tunnel: w327 -> [w339 w351 w365 w378 w391]
          frame "Open", "Standard", Default {
            w333 = T3."Standard" ("State")
            n124 = property class="VI"(reference=w339, error in=w338) -> (reference out=w336:refnum<vi>, error out=w337:errorcluster, "FP.State"=w335:T3)
            n125 = Not Equal?(x=w335, y=w333) -> (x != y?=w334:bool)
            n126 = case shown="True" w334 {
              tunnel: [w344 w346] -> w340
              tunnel: w337 -> [w343 w346]
              tunnel: w336 -> [w342 _]
              tunnel: w333 -> [w341 _]
              frame True {
                n127 = invoke class="VI" method="FP.Open"(reference=w342, error in=w343, "Activate"=TRUE, "State"=w341) -> (error out=w344:errorcluster)  [unwired: 1 in, 4 out]
              }
              frame False {
              }
            }
          }
          frame "Close", "Closed" {
            n128 = property class="VI"(reference=w351, error in=w353) -> (reference out=w350:refnum<vi>, error out=w352:errorcluster, "FP.State"=w348:T3)
            n129 = Not Equal?(x=w348, y=T3."Closed" ("Front Panel Window:State")) -> (x != y?=w347:bool)
            n130 = case shown="True" w347 {
              tunnel: [w355 w358] -> w354
              tunnel: w352 -> [w355 w357]
              tunnel: w350 -> [_ w356]
              frame False {
              }
              frame True {
                n131 = invoke class="VI" method="FP.Close"(reference=w356, error in=w357) -> (error out=w358:errorcluster)  [unwired: 1 in, 2 out]
              }
            }
          }
          frame "Hidden", "Hide" {
            w359 = T3."Hidden" ("State")
            n132 = property class="VI"(reference=w365, error in=w364) -> (reference out=w362:refnum<vi>, error out=w363:errorcluster, "FP.State"=w361:T3)
            n133 = Not Equal?(x=w361, y=w359) -> (x != y?=w360:bool)
            n134 = case shown="True" w360 {
              tunnel: [w370 w371] -> w366
              tunnel: w363 -> [w369 w371]
              tunnel: w362 -> [w368 _]
              tunnel: w359 -> [w367 _]
              frame True {
                n135 = invoke class="VI" method="FP.Open"(reference=w368, error in=w369, "State"=w367) -> (error out=w370:errorcluster)  [unwired: 2 in, 4 out]
              }
              frame False {
              }
            }
          }
          frame "Minimize", "Minimized" {
            w372 = T3."Minimized" ("State")
            n136 = property class="VI"(reference=w378, error in=w377) -> (reference out=w375:refnum<vi>, error out=w376:errorcluster, "FP.State"=w374:T3)
            n137 = Not Equal?(x=w374, y=w372) -> (x != y?=w373:bool)
            n138 = case shown="True" w373 {
              tunnel: [w383 w384] -> w379
              tunnel: w376 -> [w382 w384]
              tunnel: w375 -> [w381 _]
              tunnel: w372 -> [w380 _]
              frame True {
                n139 = invoke class="VI" method="FP.Open"(reference=w381, error in=w382, "State"=w380) -> (error out=w383:errorcluster)  [unwired: 2 in, 4 out]
              }
              frame False {
              }
            }
          }
          frame "Maximize", "Maximized" {
            w385 = T3."Maximized" ("State")
            n140 = property class="VI"(reference=w391, error in=w390) -> (reference out=w388:refnum<vi>, error out=w389:errorcluster, "FP.State"=w387:T3)
            n141 = Not Equal?(x=w387, y=w385) -> (x != y?=w386:bool)
            n142 = case shown="True" w386 {
              tunnel: [w396 w397] -> w392
              tunnel: w389 -> [w395 w397]
              tunnel: w388 -> [w394 _]
              tunnel: w385 -> [w393 _]
              frame True {
                n143 = invoke class="VI" method="FP.Open"(reference=w394, error in=w395, "State"=w393) -> (error out=w396:errorcluster)  [unwired: 2 in, 4 out]
              }
              frame False {
              }
            }
          }
        }
        n144 = call <vilib>:"Add State(s) to Queue__JKI_lib_State_Machine.vi"("State(s) in (\"\")"=w332) -> ("States Out"=w331:string)  [unwired: 14 in]
      }
      frame "UI: Change Waveform Graph Legend Num" {
        n145 = Unbundle By Name(w404) -> ("UI Refs.Data Ref"=w403:refnum<vi>)
        n146 = call "Convert API String Arguments to Data.vim"("Reference Type"=u32 0 ("Legend:Number of Rows"), "API String"=w401) -> ("error out"=w399:errorcluster, "Data"=w402:u32)  [unwired: 6 in]
        n147 = property class="WFChart (strict)"(reference=w403, error in=w399, "LegNumRows"=w402) -> (error out=w398:errorcluster)  [unwired: 1 out]
      }
      frame "UI: Update Waveform Graph" {
        n148 = call "CSM - Convert Argument to MassData.vim"("Type"=waveform(dbl)[] [] ("Data"), "MassData Argument"=w419) -> ("error out"=w417:errorcluster, "Data"=w413:waveform(dbl)[])  [unwired: 6 in]
        "WaveformGraph" <- w413
        n149 = Array Size(array=w413) -> (size(s)=w410:i32)
        n150 = feedback-in #1(w410) -> ()
        n151 = feedback #1(0) -> (w411:i32)
        n152 = Not Equal?(x=w410, y=w411) -> (x != y?=w407:bool)
        n153 = Format Into String(w410) -> (resulting string=w412:string)  [unwired: 3 in, 1 out]
        n154 = call <vilib>:"Build State String with Arguments__JKI_lib_State_Machine.vi"("Arguments (\"\")"=w412, "State"="UI: Change Waveform Graph Legend Num") -> ("State with Arguments"=w408:string)  [unwired: 4 in]
        n155 = call-poly <userlib>:"Add State(s) to Queue By BOOL++.vi"("TRUE (\"\")"=w408, "Condition"=w407, "State Queue (\"\")"=w415) -> ("Remaining States"=w416:string)  [unwired: 8 in]
      }
      frame "UI: Update AnalysisWnd 1" {
        n156 = call "CSM - Convert Argument to MassData.vim"("Type"=cluster{"f0":dbl, "df":dbl, "magnitude":dbl[]}[] [] ("FFT - (RMS)"), "MassData Argument"=w425) -> ("error out"=w424:errorcluster, "Data"=→"AnalysisWnd 1":cluster{"f0":dbl, "df":dbl, "magnitude":dbl[]}[])  [unwired: 6 in]
      }
      frame "UI: Update AnalysisWnd 2" {
        n157 = call "CSM - Convert Argument to MassData.vim"("Type"=cluster{"f0":dbl, "df":dbl, "magnitude":dbl[]}[] [] ("FFT - (RMS)"), "MassData Argument"=w432) -> ("error out"=w431:errorcluster, "Data"=→"AnalysisWnd 2":cluster{"f0":dbl, "df":dbl, "magnitude":dbl[]}[])  [unwired: 6 in]
      }
      frame "---------- Macro ----------" {
        n158 = call <vilib>:"Add State(s) to Queue__JKI_lib_State_Machine.vi"("State(s) in (\"\")"=w440) -> ("States Out"=w439:string)  [unwired: 14 in]
      }
      frame "Macro: Initialize" {
        w441 = "Data: Initialize\nInitialize Core Data\nEvents: Register\nUI: Initialize\nUI: Front Panel State >> Open\nUI: Change Waveform Graph Legend Num >> 1\nDO: Update Status >> Ready...\n\n//Permanent registrations\nAcquired Waveform@Acquisition >> API: Log@Logging -><register>\nAcquired Waveform@Acquisition >> UI: Update Waveform Graph -><register>\n\n//Dynamic registrations\nMacro: Register Analysis Relationships"  # Data: Initialize Initialize Core Data Events: Register UI: Initialize UI: Front Panel State >> Open UI: Change Waveform Graph Legend Num >> 1 DO: Update Status >> Ready...  //Permanent registrations Acquired Waveform@Acquisition >> API: Log@Logging -><register> Acquired Waveform@Acquisition >> UI: Update Waveform Graph -><register>  //Dynamic registrations Macro: Register Analysis Relationships
        # "Initialization Macro\n(This is called once, when the VI starts)"
        n159 = call <userlib>:"CSM - Populate Configuration Variables.vi"("String with INI-Variable"=w441) -> ("String"=w442:string)  [unwired: 7 in, 1 out]
        n160 = call <vilib>:"Add State(s) to Queue__JKI_lib_State_Machine.vi"("State(s) in Front (\"\")"=w442, "State(s) in (\"\")"=w447) -> ("States Out"=w446:string)  [unwired: 13 in]
      }
      frame "Macro: Register Analysis Relationships" {
        # "<2>"
        # "<1>"
        # "#CSM-NOTE\n<1> and <2> will be replaced."
        # "#CSM-NOTE\nState could be registered as status. It's similar to Status with response as its argument."
        n161 = Format Into String("Analysis Window 1") -> (resulting string=w449:string)  [unwired: 3 in, 1 out]
        n162 = Format Into String("Analysis Window 2") -> (resulting string=w448:string)  [unwired: 3 in, 1 out]
        n163 = call-poly <userlib>:"Build Message with Arguments++.vi"("States With Replace Token"="//Dynamic registrations\n\n//For AnalysisWnd 1\nAcquired Waveform@Acquisition >> API: <1>@Algorithm -><register>\nAPI: <1>@Algorithm >> UI: Update AnalysisWnd 1 -><register>\n//For AnalysisWnd 2\nAcquired Waveform@Acquisition >> API: <2>@Algorithm -><register>\nAPI: <2>@Algorithm >> UI: Update AnalysisWnd 2 -><register>" ("State(s) in Front (\"\")"), "<1>"=w449, "<2>"=w448) -> ("States"=w452:string)  [unwired: 12 in]
        n164 = Bundle By Name(cluster=w458, "Relationships"=w452) -> (w454:T9)
        n165 = call <vilib>:"Add State(s) to Queue__JKI_lib_State_Machine.vi"("State(s) in Front (\"\")"=w452, "State(s) in (\"\")"=w455) -> ("States Out"=w456:string)  [unwired: 13 in]
      }
      frame "Macro: Unregister Analysis Relationships" {
        n166 = Unbundle By Name(w470) -> ("Relationships"=w469:string)
        n167 = Search and Replace String(replace all?=TRUE ("ignore case? (F)"), case sensitive?=TRUE ("ignore case? (F)"), input string=w469, search string="<register>" ("replace string (\"\")"), replace string="<unregister>" ("replace string (\"\")")) -> (result string=w462:string)  [unwired: 3 in, 3 out]
        n168 = Bundle By Name(cluster=w470, "Relationships"="") -> (w461:T9)
        n169 = call <vilib>:"Add State(s) to Queue__JKI_lib_State_Machine.vi"("State(s) in Front (\"\")"=w462, "State(s) in (\"\")"=w463) -> ("States Out"=w464:string)  [unwired: 13 in]
      }
      frame "Macro: Start" {
        n170 = Bundle By Name(cluster=w477, "State"=UI_State."Acquiring and Logging" ("UI State")) -> (w476:T9)
        n171 = call <vilib>:"Add State(s) to Queue__JKI_lib_State_Machine.vi"("State(s) in Front (\"\")"="//Local States\nDO: Update Status >> Acquiring and Logging...\nUI: Update When Start\n\n//Send Message to Other CSM Modules\nAPI: Start -@ Logging\nAPI: Start ->| Acquisition" ("State(s) in Front (\"\")"), "State(s) in (\"\")"=w474) -> ("States Out"=w475:string)  [unwired: 13 in]
      }
      frame "Macro: Stop" {
        n172 = Unbundle By Name(w481) -> ("State"=w483:T5)
        n173 = case shown="Default" w483 {
          selector: w483 -> [w490 _]
          tunnel: [w490 UI_State."Waiting for Stop" ("UI State")] -> w482
          frame "Waiting for Exit" {
          }
          frame Default {
          }
        }
        n174 = Bundle By Name(cluster=w481, "State"=w482) -> (w487:T9)
        n175 = call <vilib>:"Add State(s) to Queue__JKI_lib_State_Machine.vi"("State(s) in Front (\"\")"="//Local States\nDO: Update Status >> Stopping...\nUI: Update When Stop\n\n//Send Message to Other CSM Modules\nAPI: Stop -@ Acquisition\nAPI: Stop -@ Logging\n" ("State(s) in Front (\"\")"), "State(s) in (\"\")"=w485) -> ("States Out"=w486:string)  [unwired: 13 in]
      }
      frame "Macro: Exit" {
        w499 = "//UI: Front Panel State >> Close"  # //UI: Front Panel State >> Close
        w496 = "//Dynamic registrations\nMacro: Unregister Analysis Relationships\n\n//Permanent registrations\nAcquired Waveform@Acquisition >> API: Log@Logging -><unregister>\nAcquired Waveform@Acquisition >> UI: Update Waveform Graph -><unregister>\n\nData: Cleanup\nEvents: Unregister\nExit"  # //Dynamic registrations Macro: Unregister Analysis Relationships  //Permanent registrations Acquired Waveform@Acquisition >> API: Log@Logging -><unregister> Acquired Waveform@Acquisition >> UI: Update Waveform Graph -><unregister>  Data: Cleanup Events: Unregister Exit
        # "Exit Macro\n(This is called once, when the VI exits)"
        n176 = Unbundle By Name(w501) -> ("Core.Close Panel on Exit?"=w500:bool)
        n177 = disable-structure shown="Enabled" {
          disable-tunnel: [w504 w516 w522] -> w493
          disable-tunnel: w492 -> [_ w515 _]
          frame Disabled {
            w511 = "Macro: Exit -@ Acquisition\nMacro: Exit -@ Logging"  # Macro: Exit -@ Acquisition Macro: Exit -@ Logging
            n178 = call <userlib>:"CSM - Module Status.vi"("CSM Name"="Algorithm") -> ("#Nodes"=w507:i32, "CSM Name (Dup)"=w509:string)  [unwired: 6 in, 3 out]
            n179 = for {
              N: w507 -> [_]
              tunnel: w509 -> [w514]
              tunnel: "Macro: Exit" -> [w513]
              tunnel: [w512] -> w505 mode=indexing
              n180 = call-poly <userlib>:"Build Message with Arguments++.vi"("State With Arguments"=w513, "Target Module (\"\")"=w514) -> ("CSM Message String"=w512:string)  [unwired: 13 in]
            }
            n181 = Build Array (concatenate)(w511, w505) -> (w506:string[])
            n182 = call <userlib>:"CSM - Compact Multiple States.vi"("Multiple States"=w506) -> ("States"=w504:string)  [unwired: 9 in]
          }
          frame Enabled {
            # "#NOTE\nHelper VI is equivalent to other case"
            n183 = call <userlib>:"CSM - List Modules.vi"() -> ("Module Names"=w518:string[])  [unwired: 10 in, 1 out]
            n184 = Search 1D Array(1D array=w518, element=w515) -> (index of element=w519:i32)  [unwired: 1 in]
            n185 = Delete From Array(array=w518, index=w519) -> (array with subset deleted=w517:string[])  [unwired: 1 in, 1 out]
            n186 = call <userlib>:"CSM - Build Exit Messages of CSMs.vi"("State With Arguments (\"Macro: Exit“)"="Macro: Exit" ("State with Arguments(\"Macro: Exit“)"), "CSMs"=w517) -> ("States"=w516:string)  [unwired: 13 in]
          }
          frame Disabled {
            # "#NOTE\nHelper VI is equivalent to other case"
            n187 = call <userlib>:"CSM - Build Exit Messages of CSMs.vi"("State With Arguments (\"Macro: Exit“)"="Macro: Exit" ("State with Arguments(\"Macro: Exit“)"), "CSMs"=string[] ["Acquisition", "Logging", "Algorithm"]) -> ("States"=w522:string)  [unwired: 13 in]
          }
        }
        n188 = Select(t=w499, s=w500, f="") -> (s? t:f=w497:string)
        n189 = call <vilib>:"Add State(s) to Queue__JKI_lib_State_Machine.vi"("State(s) in Front (\"\")"=w493, "State(s) in (\"\")"=w497, "State(s) at Back (\"\")"=w496) -> ("States Out"=w495:string)  [unwired: 12 in]
        n190 = call <vilib>:"Add State(s) to Queue__JKI_lib_State_Machine.vi"("State(s) in Front (\"\")"=w495, "State(s) in (\"\")"=w503) -> ("States Out"=w502:string)  [unwired: 13 in]
      }
      frame "---------- DoSth ----------" {
        n191 = call <vilib>:"Add State(s) to Queue__JKI_lib_State_Machine.vi"("State(s) in (\"\")"=w528) -> ("States Out"=w527:string)  [unwired: 14 in]
      }
      frame "Do: Update Status" {
        n192 = call <vilib>:"Add State(s) to Queue__JKI_lib_State_Machine.vi"("State(s) in (\"\")"=w534) -> ("States Out"=w533:string)  [unwired: 14 in]
        "Status" <- w529
      }
      frame "Do: Launch Settings Dialog" {
        # "Your code here.\n(You can make a copy of, or modify, this frame)"
        n193 = call <userlib>:"CSM - Check If Module Exists.vi"("CSM Name"="Acquisition" ("Name(\"\" to use uuid)")) -> ("error out"=w541:errorcluster, "Exist?"=w537:bool, "CSM Name (Dup)"=w539:string)  [unwired: 8 in]
        n194 = case shown="True" w537 {
          tunnel: w541 -> [w549 w561]
          tunnel: w539 -> [w545 w560]
          tunnel: w538 -> [_ w559]
          tunnel: [w548 w558] -> w536
          frame False {
            n195 = Format Into String(format string="Cannot Find the CSM which named %s !!!", w545) -> (resulting string=w544:string)  [unwired: 2 in, 1 out]
            n196 = Bundle By Name(cluster=w549, "status"=TRUE, "source"=w544) -> (w548:errorcluster)
          }
          frame True {
            w553 = T3."Standard" ("State")
            n197 = call <userlib>:"CSM - Module VI Reference.vi"("Current Module (\"\" to Generate an ID)"=w559, "error in (no error)"=w561, "Force? (F)"=TRUE ("force?(F)"), "CSM Name"=w560) -> ("error out"=w551:errorcluster, "CSM Module VIRef"=w552:refnum<vi>)  [unwired: 6 in]
            n198 = property class="VI"(reference=w552, error in=w551) -> (reference out=w556:refnum<vi>, error out=w557:errorcluster, "FP.State"=w555:T3)
            n199 = Not Equal?(x=w555, y=w553) -> (x != y?=w554:bool)
            n200 = case shown="True" w554 {
              tunnel: [w568 w570] -> w558
              tunnel: w557 -> [w563 w570]
              tunnel: w556 -> [w562 _]
              tunnel: w553 -> [w567 _]
              frame True {
                n201 = property class="VI"(reference=w562, error in=w563, "FP.Behavior"=T6."Modal" ("Front Panel Window:Behavior")) -> (reference out=w565:refnum<vi>, error out=w566:errorcluster)
                n202 = invoke class="VI" method="FP.Open"(reference=w565, error in=w566, "Activate"=TRUE, "State"=w567) -> (error out=w568:errorcluster)  [unwired: 1 in, 4 out]
              }
              frame False {
              }
            }
          }
        }
      }
      frame "Do: Confirm Quit" {
        n203 = Unbundle By Name(w575) -> ("State"=w578:T5)
        n204 = case shown="\"Acquiring and Logging\"" w578 {
          tunnel: [UI_State."Idle" ("UI State") w587] -> w577
          tunnel: w575 -> [w582 w586]
          tunnel: [w582 w585] -> w576
          tunnel: [TRUE w584] -> w571
          frame Default {
          }
          frame "Acquiring and Logging" {
            n205 = Two Button Dialog(message="Are you sure you want to quit while the acquisition is running?" ("Confirm Quit Message"), 1:"No" ("No"), 2:"Yes" ("Yes")) -> (T button?=w588:bool)
            n206 = case shown="False" w588 {
              tunnel: [UI_State."Acquiring and Logging" ("UI State") UI_State."Waiting for Exit" ("UI State")] -> w587
              tunnel: w586 -> [w592 w595]
              tunnel: [w592 w595] -> w585
              tunnel: [_ TRUE] -> w584
              frame False {
                # "User did not want to quit."
              }
              frame True {
              }
            }
          }
        }
        n207 = Bundle By Name(cluster=w576, "State"=w577) -> (w574:T9)
        n208 = call-poly <userlib>:"Add State(s) to Queue By BOOL++.vi"("TRUE (\"\")"="Macro: Exit", "Condition"=w571, "State Queue (\"\")"=w580) -> ("Remaining States"=w573:string)  [unwired: 8 in]
      }
    }
  }
  n209 = call <userlib>:"CSM - Sync Configuration Variables to File.vi"("All Temp Variable to Default Ini(F)"=TRUE, "error in (no error)"=w2) -> ("error out"=w1:errorcluster)  [unwired: 7 in]
  n210 = disable-structure shown="RUN_TIME_ENGINE==True" {
    disable-tunnel: w1 -> [_ _]
    frame condition #0 (active) {
    }
    frame condition #1 {
      n211 = Quit LabVIEW(quit? (T)=TRUE) -> ()
    }
  }
